vi "_test_dll.vi"() -> ()   [LabVIEW 2019]
uses:
  BRC-DAQ.lvlib
  Public/brc_daq_pModuleInfo.ctl
panel:
  in  "rawValue":bool
  out "Waveform Graph":waveform(dbl)[](graph)
  out "Numeric":i32
  in  "stop":bool
  out "error out":errorcluster
  out "current":dbl
  out "coupling_mode":i32
  out "sample_rate":i32
  out "Array":T1[](array[typedef])
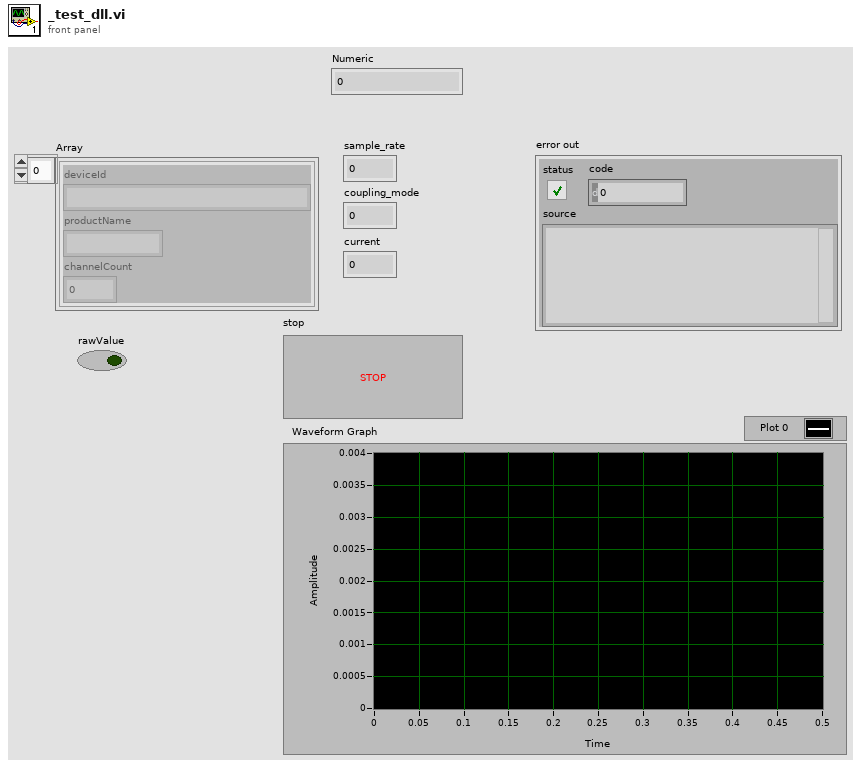
[diagram p1: front panel]
types:
  T1 = typedef "BRC-DAQ.lvlib/brc_daq_pModuleInfo.ctl" = cluster{"deviceId":string, "productName":string, "channelCount":i32}
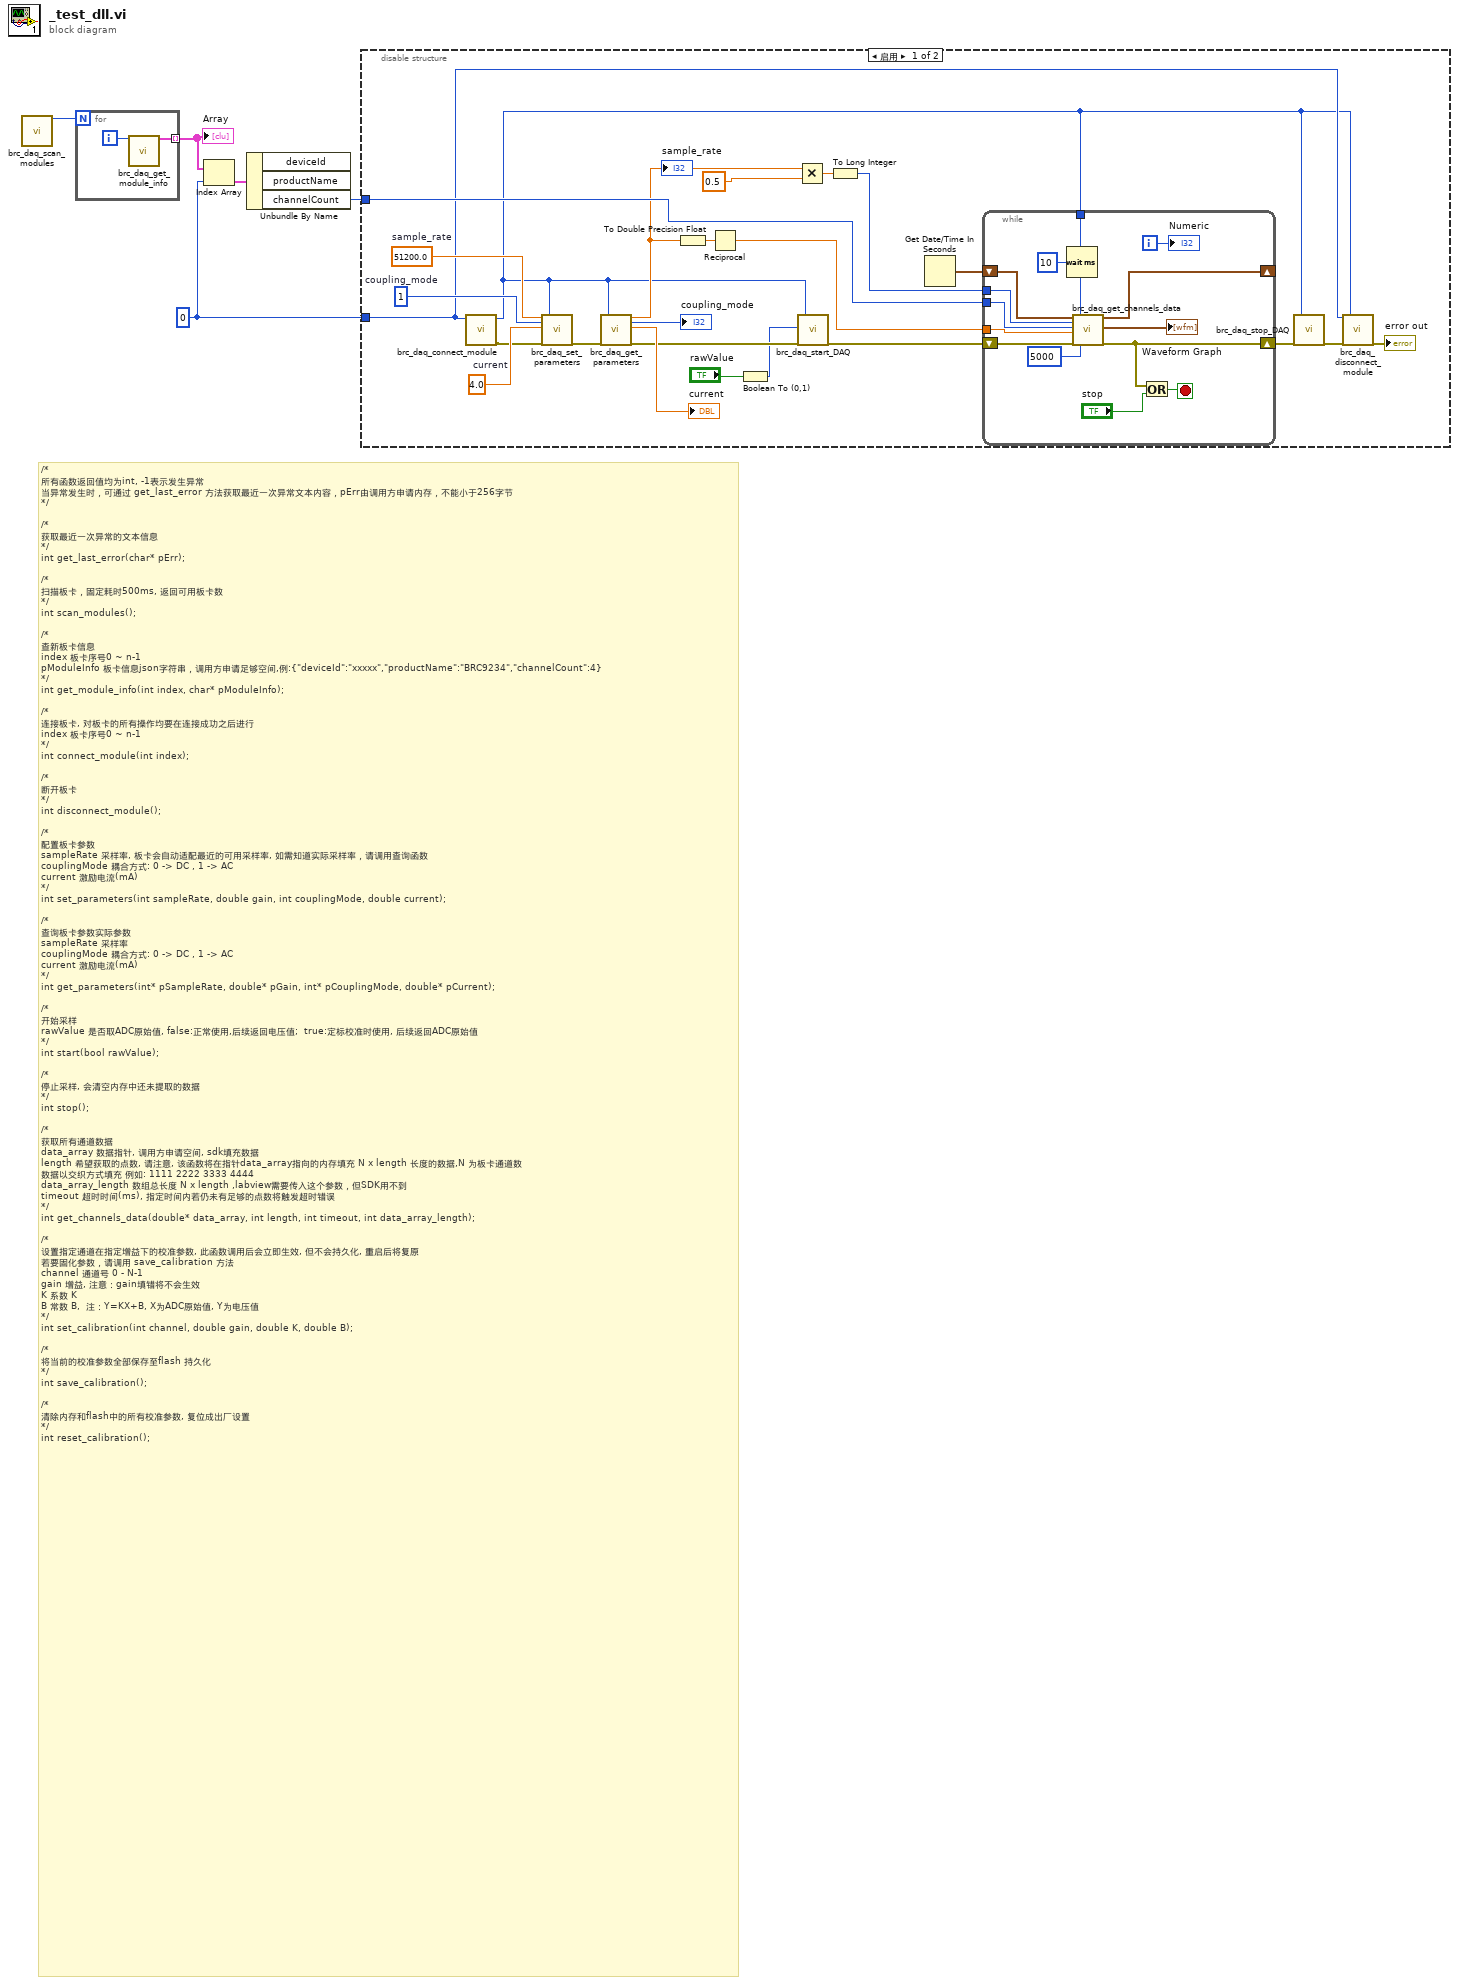
[diagram p0: block diagram]
diagram:
  w1 = 0 ("index")
  # "/*\n所有函数返回值均为int, -1表示发生异常\n当异常发生时，可通过 get_last_error 方法获取最近一次异常文本内容，pErr由调用方申请内存，不能小于256字节\n*/\n\n/*\n获取最近一次异常的文本信息\n*/\nint get_last_error(char* pErr);\n\n/*\n扫描板卡，固定耗时500ms, 返回可用板卡数\n*/\nint scan_modules();\n\n/*\n查新板卡信息\nindex 板卡序号0 ~ n-1\npModuleInfo 板卡信息json字符串，调用方申请足够空间,例:{\"deviceId\":\"xxxxx\",\"productName\":\"BRC9234\",\"channelCount\":4}\n*/\nint get_module_info(int index, char* pModuleInfo);\n\n/*\n连接板卡, 对板卡的所有操作均要在连接成功之后进行\nindex 板卡序号0 ~ n-1\n*/\nint connect_module(int index);\n\n/*\n断开板卡\n*/\nint disconnect_module();\n\n/*\n配置板卡参数\nsampleRate 采样率, 板卡会自动适配最近的可用采样率, 如需知道实际采样率，请调用查询函数\ncouplingMode 耦合方式: 0 -> DC , 1 -> AC\ncurrent 激励电流(mA)\n*/\nint set_parameters(int sampleRate, double gain, int couplingMode, double current);\n\n/*\n查询板卡参数实际参数\nsampleRate 采样率\ncouplingMode 耦合方式: 0 -> DC , 1 -> AC\ncurrent 激励电流(mA)\n*/\nint get_parameters(int* pSampleRate, double* pGain, int* pCouplingMode, double* pCurrent);\n\n/*\n开始采样\nrawValue 是否取ADC原始值, false:正常使用,后续返回电压值;  true:定标校准时使用, 后续返回ADC原始值\n*/\nint start(bool rawValue);\n\n/*\n停止采样, 会清空内存中还未提取的数据\n*/\nint stop();\n\n/*\n获取所有通道数据\ndata_array 数据指针, 调用方申请空间, sdk填充数据\nlength 希望获取的点数, 请注意, 该函数将在指针data_array指向的内存填充 N x length 长度的数据,N 为板卡通道数\n数据以交织方式填充 例如: 1111 2222 3333 4444\ndata_array_length 数组总长度 N x length ,labview需要传入这个参数，但SDK用不到\ntimeout 超时时间(ms), 指定时间内若仍未有足够的点数将触发超时错误\n*/\nint get_channels_data(double* data_array, int length, int timeout, int data_array_length);\n\n/*\n设置指定通道在指定增益下的校准参数, 此函数调用后会立即生效, 但不会持久化, 重启后将复原\n若要固化参数，请调用 save_calibration 方法\nchannel 通道号 0 - N-1\ngain 增益, 注意：gain填错将不会生效\nK 系数 K\nB 常数 B,  注：Y=KX+B, X为ADC原始值, Y为电压值\n*/\nint set_calibration(int channel, double gain, double K, double B);\n\n/*\n将当前的校准参数全部保存至flash 持久化\n*/\nint save_calibration();\n\n/*\n清除内存和flash中的所有校准参数, 复位成出厂设置\n*/\nint reset_calibration();"
  n1 = call "brc_daq_scan_modules.vi"() -> ("module_number"=w2:i32)  [unwired: 18 in, 1 out]
  n2 = for {
    N: w2 -> [_]
    tunnel: [w7] -> w4 mode=indexing
    i -> [w6]
    n3 = call "brc_daq_get_module_info.vi"("index"=w6) -> ("pModuleInfo_cluster"=w7:T1)  [unwired: 17 in, 1 out]
  }
  "Array" <- w4
  n4 = Index Array(array=w4, index=w1) -> (element=w3:T1)
  n5 = Unbundle By Name(w3) -> ("channelCount"=w5:i32)  [unwired: 2 out]
  n6 = disable-structure shown="启用" {
    disable-tunnel: w1 -> [w10 _]
    disable-tunnel: w5 -> [w31 _]
    frame Enabled {
      w25 = 4.0  # current
      w24 = 1  # coupling_mode
      w23 = 51200.0  # sample_rate
      n7 = call "brc_daq_connect_module.vi"("index"=w10) -> ("error out"=w8:errorcluster, "return_value"=w9:i32)  [unwired: 9 in]
      n8 = call "brc_daq_set_parameters.vi"("sample_rate"=w23, "coupling_mode"=w24, "current_mA"=w25, "error in (no error)"=w8, "mHandle"=w9) -> ("error out"=w19:errorcluster)  [unwired: 14 in]
      n9 = call "brc_daq_get_parameters.vi"("error in (no error)"=w19, "mHandle"=w9) -> ("sample_rate"=w22:dbl, "coupling_mode"=→"coupling_mode":i32, "current"=→"current":dbl, "error out"=w18:errorcluster)  [unwired: 14 in]
      "sample_rate" <- w22
      n10 = To Double Precision Float(number=w22) -> (double precision float=w27:dbl)
      n11 = Reciprocal(x=w27) -> (1/x=w26:dbl)
      n12 = Boolean To (0,1)(Boolean="rawValue") -> (0, 1=w11:i16)
      n13 = Multiply(x=w22, y=0.5) -> (x*y=w30:dbl)
      n14 = call "brc_daq_start_DAQ.vi"("rawValue"=w11, "error in (no error)"=w18, "mHandle"=w9) -> ("error out"=w17:errorcluster)  [unwired: 16 in]
      n15 = To Long Integer(number=w30) -> (32bit integer=w29:i32)
      n16 = Get Date/Time In Seconds() -> (seconds since 1Jan1904=w13:timestamp)
      n17 = while {
        shift-right: [w43] -> w16
        shift-left: w17 -> [w45]
        tunnel: w29 -> [w42]
        tunnel: w31 -> [w41]
        tunnel: w26 -> [w38]
        shift-right: [w34] -> _
        shift-left: w13 -> [w36]
        tunnel: w9 -> [w33]
        i -> [w37]
        stop <- w44 stop-if-true
        n18 = Wait (ms)(milliseconds to wait=u32 10) -> ()  [unwired: 1 out]
        n19 = call "brc_daq_get_channels_data.vi"("t0_in"=w36, "samples_per_ch"=w42, "ch_number"=w41, "dt"=w38, "error in (no error)"=w45, "mHandle"=w33, "time_out_ms"=5000) -> ("t0_out"=w34:timestamp, "data_out"=→"Waveform Graph":waveform(dbl)[], "error out"=w43:errorcluster)  [unwired: 10 in]
        n20 = Or(x=w43, y="stop") -> (x .or. y?=w44:bool)
        "Numeric" <- w37
      }
      n21 = call "brc_daq_stop_DAQ.vi"("error in (no error)"=w16, "mHandle"=w9) -> ("error out"=w15:errorcluster)  [unwired: 17 in]
      n22 = call "brc_daq_disconnect_module.vi"("index"=w10, "error in (no error)"=w15, "mHandle"=w9) -> ("error out"=→"error out":errorcluster)  [unwired: 16 in]
    }
    frame Disabled {
    }
  }
